vi "Array Transform.vi"(0 "input array":dbl[][](array[numeric])) -> (14 "vertical flip":dbl[][](array[numeric]), 15 "horizontal flip":dbl[][](array[numeric]), 16 "rotate 90":dbl[][](array[numeric]), 17 "rotate 180":dbl[][](array[numeric]), 18 "rotate 270":dbl[][](array[numeric]), 19 "diagonal flip (inverse)":dbl[][](array[numeric]))   [LabVIEW 2013]
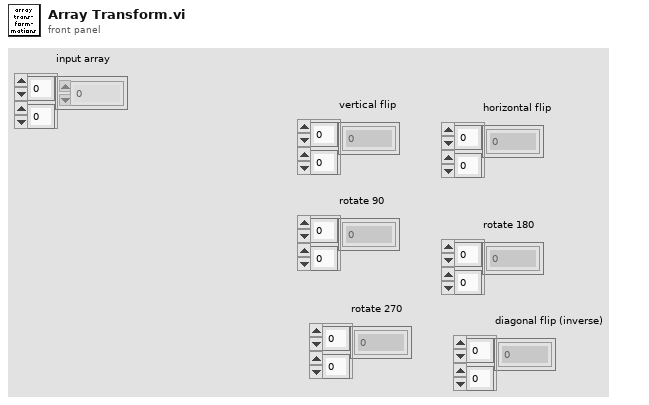
[diagram p1: front panel]
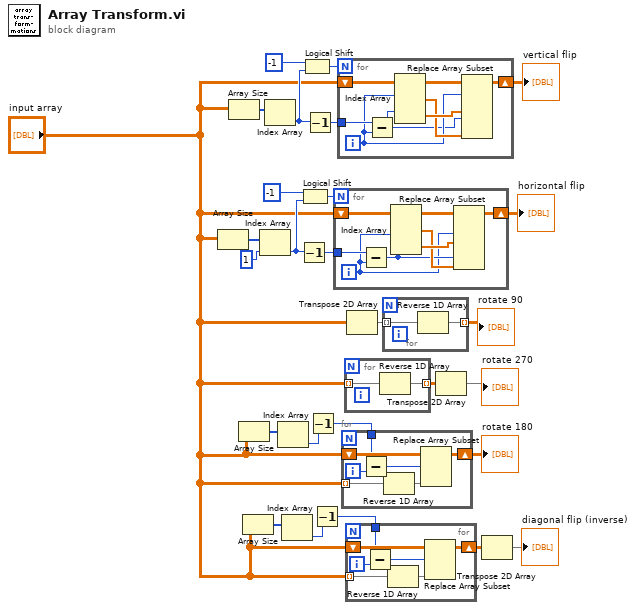
[diagram p0: block diagram]
diagram:
  n1 = Array Size(array="input array") -> (size(s)=w17:i32[])
  n2 = Array Size(array="input array") -> (size(s)=w26:i32[])
  n3 = Array Size(array="input array") -> (size(s)=w14:i32[])
  n4 = Array Size(array="input array") -> (size(s)=w9:i32[])
  n5 = Index Array(array=w17, index=1) -> (element=w19:i32)
  n6 = Index Array(array=w26) -> (element=w24:i32)  [unwired: 1 in]
  n7 = Index Array(array=w14) -> (element=w12:i32)  [unwired: 1 in]
  n8 = Index Array(array=w9) -> (element=w11:i32)  [unwired: 1 in]
  n9 = Decrement(x=w19) -> (x-1=w21:i32)
  n10 = Logical Shift(y=i8 -1, x=w19) -> (x << y=w18:i32)
  n11 = Logical Shift(y=i8 -1, x=w24) -> (x << y=w25:i32)
  n12 = Decrement(x=w24) -> (x-1=w22:i32)
  n13 = Decrement(x=w12) -> (x-1=w13:i32)
  n14 = Decrement(x=w11) -> (x-1=w10:i32)
  n15 = for {
    N: w18 -> [_]
    shift-right: [w34] -> w5
    shift-left: "input array" -> [w33]
    tunnel: w21 -> [w30]
    i -> [w28]
    n16 = Subtract(x=w30, y=w28) -> (x-y=w29:i32)
    n17 = Index Array(array=w33, index (col) #1=w28, index (col) #2=w29) -> (element #1=w31:dbl[], element #2=w32:dbl[])  [unwired: 2 in]
    n18 = Replace Array Subset(array=w33, new element #1=w32, index (col) #1=w28, new element #2=w31, index (col) #2=w29) -> (w34:dbl[][])  [unwired: 2 in]
  }
  "horizontal flip" <- w5
  n19 = for {
    N: w25 -> [_]
    shift-right: [w41] -> w6
    shift-left: "input array" -> [w40]
    tunnel: w22 -> [w37]
    i -> [w36]
    n20 = Subtract(x=w37, y=w36) -> (x-y=w35:i32)
    n21 = Index Array(array=w40, index (row) #1=w36, index (row) #2=w35) -> (element #1=w38:dbl[], element #2=w39:dbl[])  [unwired: 2 in]
    n22 = Replace Array Subset(array=w40, new element #1=w39, index (row) #1=w36, new element #2=w38, index (row) #2=w35) -> (w41:dbl[][])  [unwired: 2 in]
  }
  "vertical flip" <- w6
  n23 = for {
    shift-right: [w48] -> w2
    shift-left: "input array" -> [w47]
    tunnel: w13 -> [w45]
    tunnel: "input array" -> [w42] mode=indexing
    i -> [w46]
    n24 = Subtract(x=w45, y=w46) -> (x-y=w44:i32)
    n25 = Reverse 1D Array(array=w42) -> (reversed array=w43:dbl[])
    n26 = Replace Array Subset(array=w47, new element=w43, index (row)=w44) -> (w48:dbl[][])  [unwired: 1 in]
  }
  "rotate 180" <- w2
  n27 = for {
    tunnel: "input array" -> [w50] mode=indexing
    tunnel: [w49] -> w27 mode=indexing
    n28 = Reverse 1D Array(array=w50) -> (reversed array=w49:dbl[])
  }
  n29 = for {
    shift-right: [w57] -> w8
    shift-left: "input array" -> [w56]
    tunnel: w10 -> [w54]
    tunnel: "input array" -> [w51] mode=indexing
    i -> [w55]
    n30 = Subtract(x=w54, y=w55) -> (x-y=w53:i32)
    n31 = Reverse 1D Array(array=w51) -> (reversed array=w52:dbl[])
    n32 = Replace Array Subset(array=w56, new element=w52, index (row)=w53) -> (w57:dbl[][])  [unwired: 1 in]
  }
  n33 = Transpose 2D Array(2D array="input array") -> (transposed array=w16:dbl[][])
  n34 = for {
    tunnel: w16 -> [w59] mode=indexing
    tunnel: [w58] -> w4 mode=indexing
    n35 = Reverse 1D Array(array=w59) -> (reversed array=w58:dbl[])
  }
  "rotate 90" <- w4
  n36 = Transpose 2D Array(2D array=w27) -> (transposed array=→"rotate 270":dbl[][])
  n37 = Transpose 2D Array(2D array=w8) -> (transposed array=→"diagonal flip (inverse)":dbl[][])
